vi "Get Switch Heat.vi"(8 "error in (no error)":errorcluster, 11 "Instrument.1820 in":refnum<class "Instrument.Oxford1820.lvclass">) -> (0 "error out":errorcluster, 1 "Heater On?":bool, 2 "Switch Heater Status":string, 3 "Instrument.1820 in":refnum<class "Instrument.Oxford1820.lvclass">)   [LabVIEW 2019, in "Instrument.Oxford1820.lvclass"]
uses:
  Instrument.Oxford1820.lvclass
  551bc44b-60b2-42e1-9da9-ee101d7c4bc7.vi
  Typedefs/Instrument.Oxford1820.protectedCommands-enum.ctl
  C:/Program Files/National Instruments/LabVIEW 2019/user.lib/LevyLab/Instrument Framework/Instrument Types/Cryostat/Instrument.Cryostat.lvclass
  C:/Program Files/National Instruments/LabVIEW 2019/user.lib/LevyLab/Instrument Framework/Instrument/Instrument.lvclass
  C:/Program Files/National Instruments/LabVIEW 2019/vi.lib/JKI/JKI SMO/SMO/SMO.lvclass
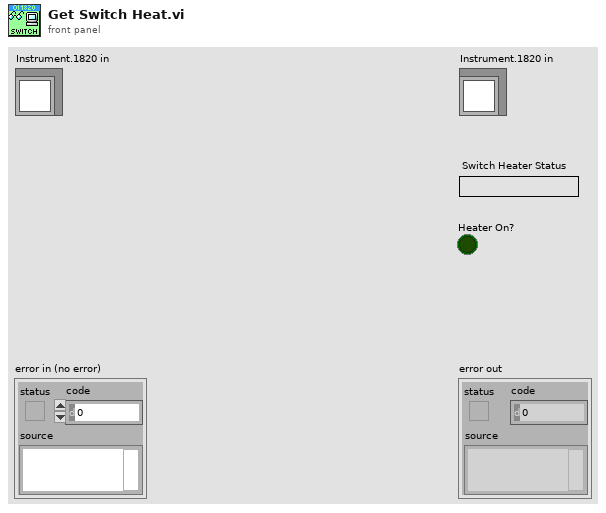
[diagram p1: front panel]
types:
  T1 = typedef "Instrument.Oxford1820.lvclass/Instrument.Oxford1820.protectedCommands-enum.ctl" = enum16{"setAction", "setTarget", "setSwitchHeat", "setLambda", "setFillMode", "setNeedleValve", "getStatus", "getTarget", "getSwitchHeat", "getPSUField", "setSequenceStatus"}
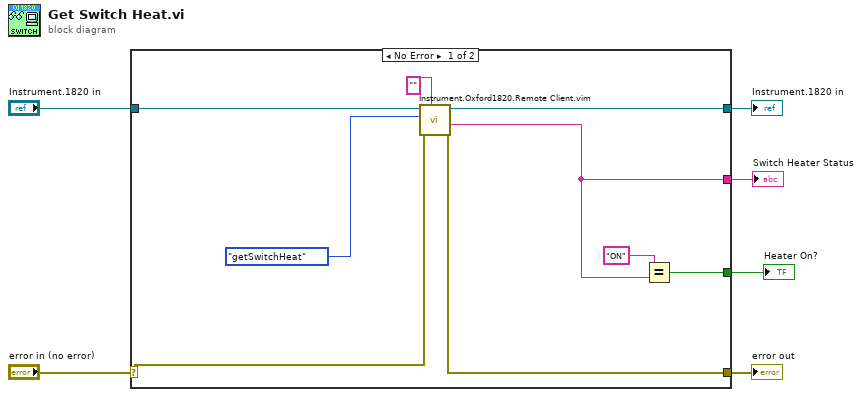
[diagram p0: block diagram]
diagram:
  n1 = case shown="No Error" "error in (no error)" {
    selector: "error in (no error)" -> [w13 w17]
    tunnel: [w10 w17] -> w5
    tunnel: [w9 w16] -> w3
    tunnel: "Instrument.1820 in" -> [w12 w16]
    tunnel: [w11 _] -> w2
    tunnel: [w14 _] -> w1
    frame No Error {
      n2 = call "Instrument.Oxford1820.Remote Client.vim"("Data Out type"="", "error in (no error)"=w13, "Commands"=Instrument.Oxford1820.protectedCommands-enum."getSwitchHeat", "Instrument.1820 in"=w12) -> ("error out"=w10:errorcluster, "Data out"=w11:string, "Instrument.1820 out"=w9:refnum<class "Instrument.Oxford1820.lvclass">)  [unwired: 5 in]
      n3 = Equal?(x="ON", y=w11) -> (x = y?=w14:bool)
    }
    frame Error {
    }
  }
  "error out" <- w5
  "Instrument.1820 in" <- w3
  "Switch Heater Status" <- w2
  "Heater On?" <- w1
